vi "Schedule Editor.vi"() -> ()   [LabVIEW 2023]
uses:
  Schedule.ctl
  Tubes.ctl
panel:
  in  "Tube Type":T1
  in  "Schedule":T2
  in  "Schedule Filename":string
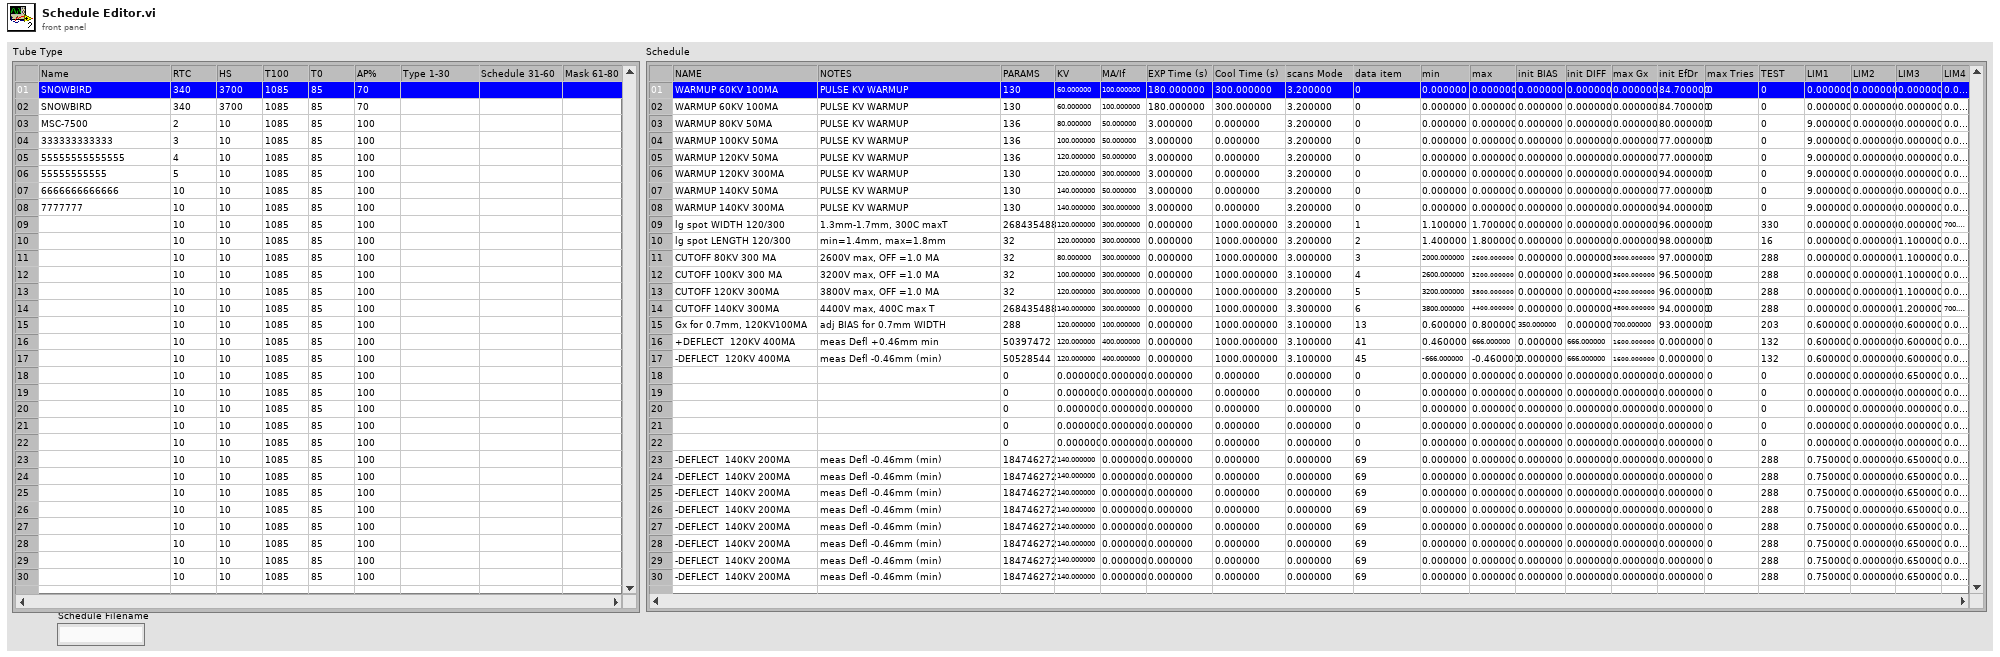
[diagram p1: front panel]
types:
  T1 = typedef "Tubes.ctl" = i32
  T2 = typedef "Schedule.ctl" = i32
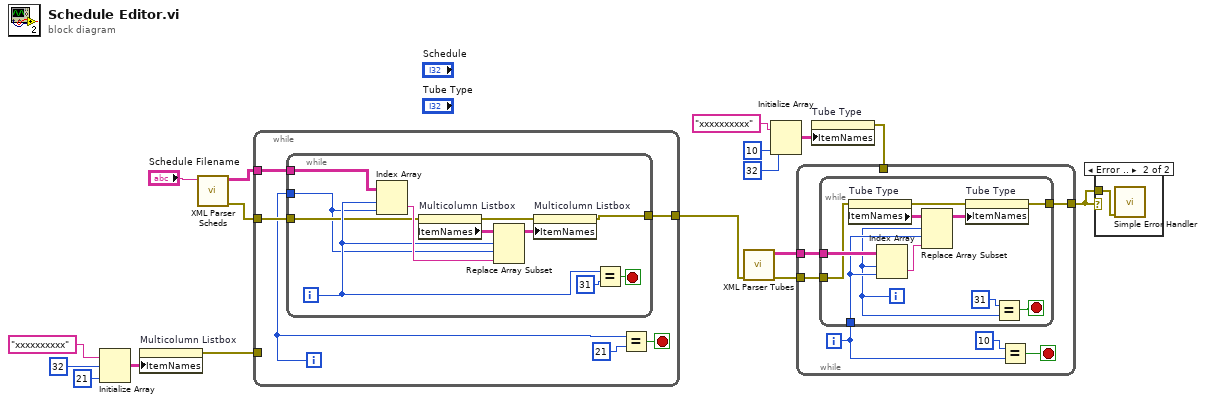
[diagram p0: block diagram]
diagram:
  n1 = Initialize Array("xxxxxxxxxx", 32 ("dimension size"), 21 ("dimension size")) -> (w10:string[][])
  n2 = property on="Multicolumn Listbox" class="MCListbox (strict)"("ItemNames"=w10) -> (error out=w14:errorcluster)  [unwired: 2 in, 1 out]
  n3 = call "XML Parser Scheds.vi"("Schedule Filename"="Schedule Filename") -> ("error out"=w15:errorcluster, "output array"=w16:string[][])  [unwired: 9 in]
  n4 = while {
    tunnel: w16 -> [w21]
    tunnel: w15 -> [w20]
    tunnel: [w19] -> w3
    tunnel: w14 -> [_]
    i -> [w18]
    stop <- w22 stop-if-true
    n5 = while {
      tunnel: w18 -> [w24]
      tunnel: w21 -> [w32]
      tunnel: w20 -> [w29]
      tunnel: [w26] -> w19
      i -> [w30]
      stop <- w33 stop-if-true
      n6 = Index Array(array=w32, index (row)=w30, index (col)=w24) -> (element=w31:string)
      n7 = property on="Multicolumn Listbox" class="MCListbox (strict)"(error in=w29) -> (error out=w27:errorcluster, "ItemNames"=w28:string[][])  [unwired: 1 in, 1 out]
      n8 = Replace Array Subset(array=w28, new element=w31, index (row)=w30, index (col)=w24) -> (w25:string[][])
      n9 = property on="Multicolumn Listbox" class="MCListbox (strict)"(error in=w27, "ItemNames"=w25) -> (error out=w26:errorcluster)  [unwired: 1 in, 1 out]
      n10 = Equal?(x=w30, y=31) -> (x = y?=w33:bool)
    }
    n11 = Equal?(x=w18, y=21) -> (x = y?=w22:bool)
  }
  n12 = call "XML Parser Tubes.vi"("error in (no error)"=w3) -> ("error out"=w4:errorcluster, "output array"=w5:string[][])  [unwired: 9 in]
  n13 = Initialize Array("xxxxxxxxxx", 32 ("dimension size"), 10 ("dimension size")) -> (w6:string[][])
  n14 = property on="Tube Type" class="MCListbox (strict)"("ItemNames"=w6) -> (error out=w2:errorcluster)  [unwired: 2 in, 1 out]
  n15 = while {
    tunnel: w5 -> [w38]
    tunnel: [w36] -> w1
    tunnel: w4 -> [w35]
    tunnel: w2 -> [_]
    i -> [w37]
    stop <- w39 stop-if-true
    n16 = while {
      tunnel: w38 -> [w47]
      tunnel: w37 -> [w45]
      tunnel: [w43] -> w36
      tunnel: w35 -> [w41]
      i -> [w44]
      stop <- w50 stop-if-true
      n17 = property on="Tube Type" class="MCListbox (strict)"(error in=w41) -> (error out=w42:errorcluster, "ItemNames"=w49:string[][])  [unwired: 1 in, 1 out]
      n18 = Index Array(array=w47, index (row)=w44, index (col)=w45) -> (element=w46:string)
      n19 = Replace Array Subset(array=w49, new element=w46, index (row)=w44, index (col)=w45) -> (w48:string[][])
      n20 = property on="Tube Type" class="MCListbox (strict)"(error in=w42, "ItemNames"=w48) -> (error out=w43:errorcluster)  [unwired: 1 in, 1 out]
      n21 = Equal?(x=31, y=w44) -> (x = y?=w50:bool)
    }
    n22 = Equal?(x=10, y=w37) -> (x = y?=w39:bool)
  }
  n23 = case shown="Error .." w1 {
    tunnel: w1 -> [_ w52]
    frame No Error {
    }
    frame Error {
      n24 = call <vilib>:"Simple Error Handler.vi"("error in (no error)"=w52) -> ()  [unwired: 4 in, 5 out]
    }
  }
